vi "mini_test_app.vi"() -> ()   [LabVIEW 2015]
doc: "Mini test app"
uses:
  <vilib>/Utility/error.llb/DialogType.ctl
  Type Definitions/Highway_Data_Control.ctl
panel:
  out "GB ID":string="\r\n" caption="GB Instrument ID"
  out "Hi-Pot ID":string="\r\n" caption="Hi-Pot Instrument ID"
  out "I/F type":string caption="Interface type"
  out "Results GB":string
  out "Status GB":string
  in  "Stop GB":bool
  in  "Start GB":bool
  in  "Stop HiPot":bool
  out "Results HP":string
  in  "Exit Button":bool
  in  "Start HiPot":bool
  out "Status HP":string
  # "Warning. This app is a proof of concept and has no other purpose, \nit is not intended for production. Likewise, it has no error handling. \nUse at your own risk."
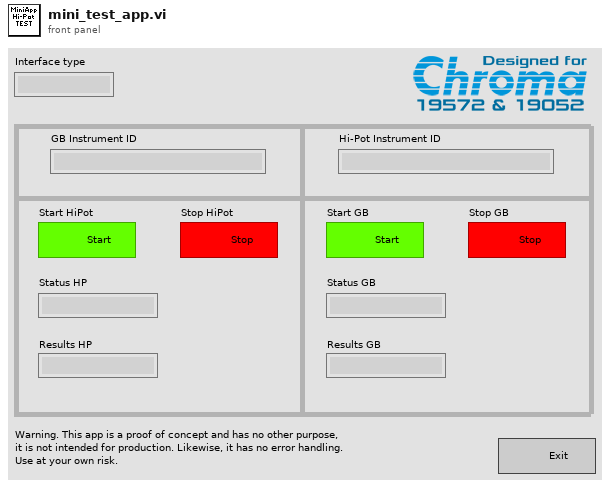
[diagram p1: front panel]
types:
  T1 = typedef "Highway_Data_Control.ctl" = cluster{"Status HP":string, "Results HP":string, "Status GB":string, "Results GB":string}
  T2 = typedef "DialogType.ctl" = u16
  T3 = cluster{"VISA1 Inst ID":string, "VISA2 Inst ID":string, "I/F type":string}
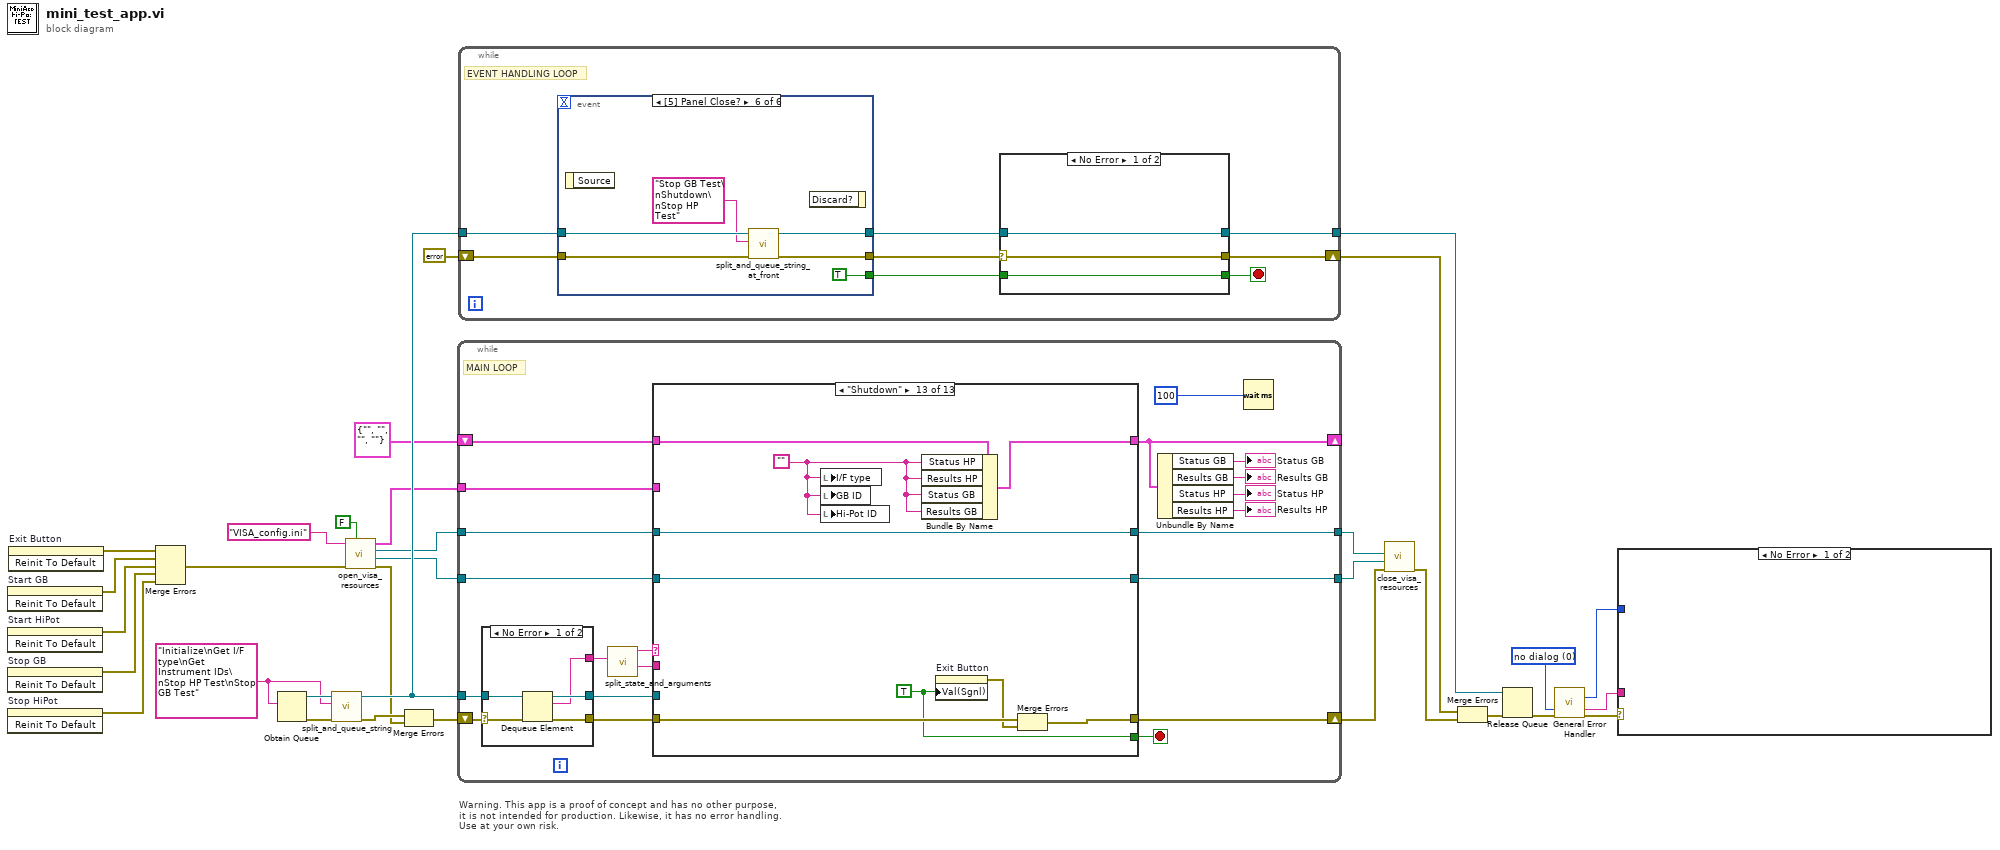
[diagram p0: block diagram]
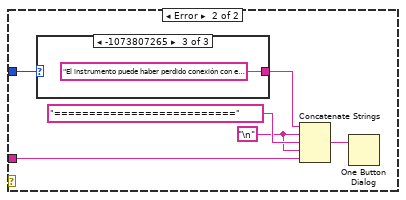
[diagram p2: hidden frame]
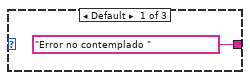
[diagram p3: hidden frame]
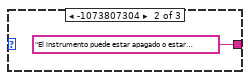
[diagram p4: hidden frame]
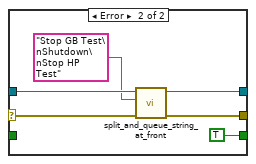
[diagram p5: hidden frame]
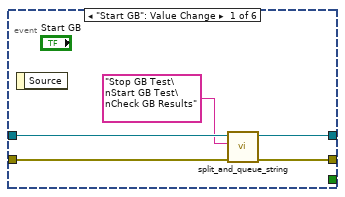
[diagram p6: hidden frame]
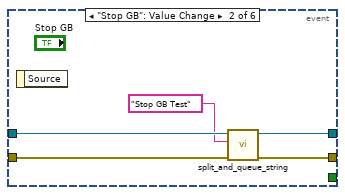
[diagram p7: hidden frame]
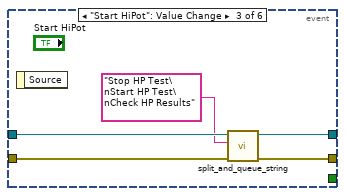
[diagram p8: hidden frame]
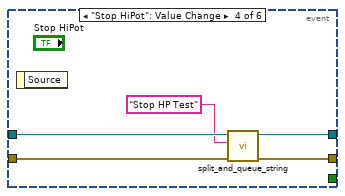
[diagram p9: hidden frame]
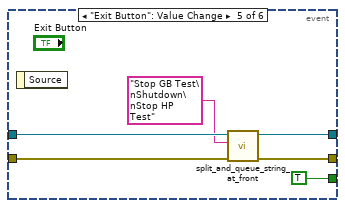
[diagram p10: hidden frame]
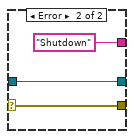
[diagram p11: hidden frame]
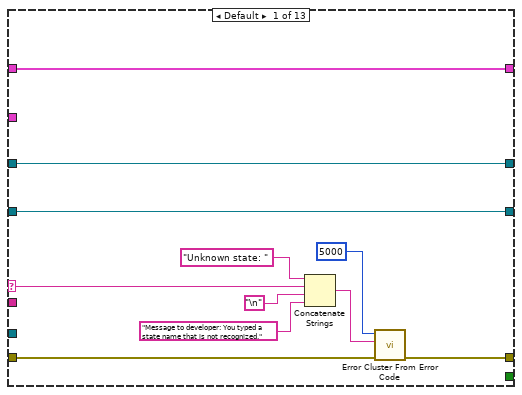
[diagram p12: hidden frame]
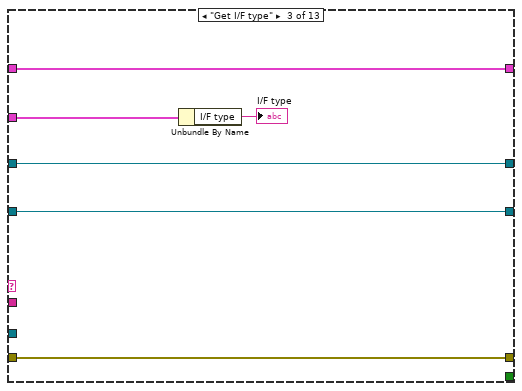
[diagram p14: hidden frame]
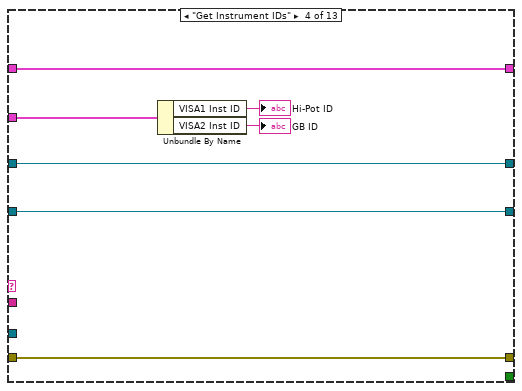
[diagram p15: hidden frame]
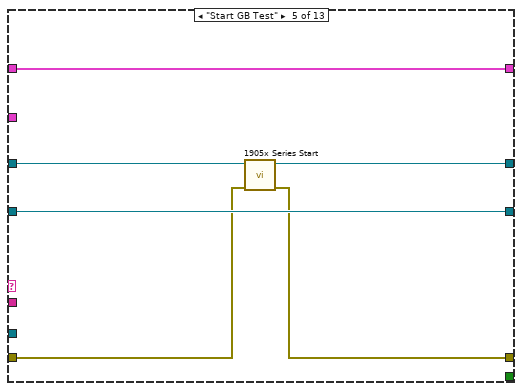
[diagram p16: hidden frame]
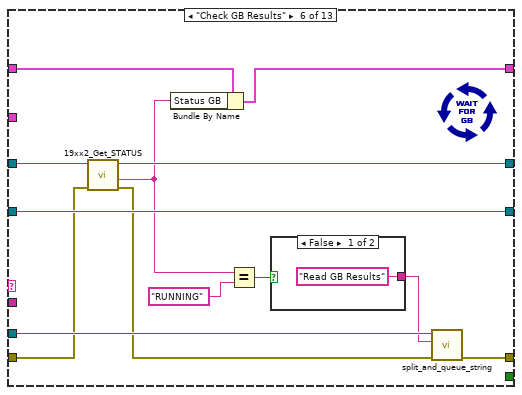
[diagram p17: hidden frame]
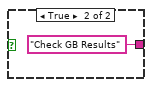
[diagram p18: hidden frame]
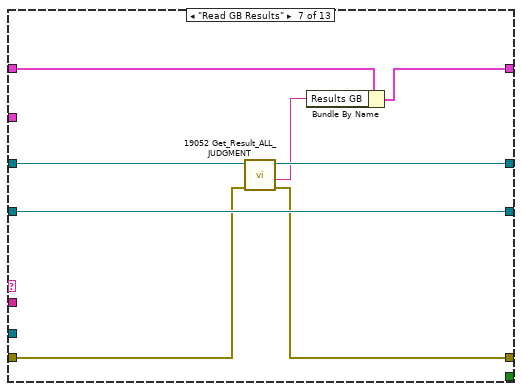
[diagram p19: hidden frame]
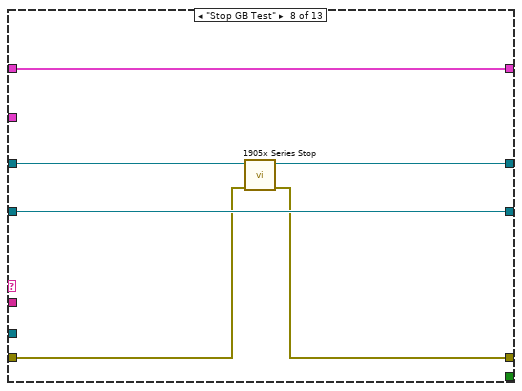
[diagram p20: hidden frame]
diagram:
  w13 = T2 0 items=["no dialog", "OK message", "continue or stop message", "OK message + warnings", "continue/stop + warnings"] ("type of dialog (OK msg:1)")
  w26 = "Initialize\nGet I/F type\nGet Instrument IDs\nStop HP Test\nStop GB Test" ("program string")
  # "Warning. This app is a proof of concept and has no other purpose, \nit is not intended for production. Likewise, it has no error handling. \nUse at your own risk."
  n1 = invoke on="Start GB" class="Bool" method="Reinit To Default"() -> (error out=w5:errorcluster)  [unwired: 3 in, 2 out]
  n2 = invoke on="Start HiPot" class="Bool" method="Reinit To Default"() -> (error out=w4:errorcluster)  [unwired: 3 in, 2 out]
  n3 = invoke on="Stop GB" class="Bool" method="Reinit To Default"() -> (error out=w3:errorcluster)  [unwired: 3 in, 2 out]
  n4 = invoke on="Stop HiPot" class="Bool" method="Reinit To Default"() -> (error out=w2:errorcluster)  [unwired: 3 in, 2 out]
  n5 = invoke on="Exit Button" class="Bool (strict)" method="Reinit To Default"() -> (error out=w7:errorcluster)  [unwired: 3 in, 2 out]
  n6 = Merge Errors(w7, w5, w4, w3, w2) -> (w6:errorcluster)
  n7 = Obtain Queue(element data type=w26) -> (queue out=w32:refnum<queue>, error out=w31:errorcluster)  [unwired: 4 in, 1 out]
  n8 = call "split_and_queue_string.vi"("error in (no error)"=w31, "program string"=w26, "queue in"=w32) -> ("error out"=w25:errorcluster, "queue out"=w24:refnum<queue>)  [unwired: 7 in]
  n9 = call "open_visa_resources.vi"("test mode"=FALSE, "error in (no error)"=w6, "config file in"="VISA_config.ini") -> ("error out"=w17:errorcluster, "VISA resource name for 19052"=w16:refnum<visa-resource-name>, "VISA resource name for 19572"=w9:refnum<visa-resource-name>, "Assgs"=w15:T3)  [unwired: 5 in]
  n10 = Merge Errors(w25, w17) -> (w18:errorcluster)
  n11 = while {
    shift-right: [w51] -> w21
    shift-left: w18 -> [w39]
    tunnel: w24 -> [w40]
    tunnel: w15 -> [w44]
    tunnel: w16 -> [w47]
    tunnel: [w46] -> w22
    tunnel: w9 -> [w43]
    tunnel: [w42] -> w8
    shift-right: [w37] -> _
    shift-left: T1 {"Status HP"="", "Results HP"="", "Status GB"="", "Results GB"=""} -> [w38]
    stop <- w45 stop-if-true
    # "MAIN LOOP"
    n12 = case shown="No Error" w39 {
      selector: w39 -> [w58 w61]
      tunnel: [w57 w61] -> w52
      tunnel: w40 -> [w54 w60]
      tunnel: [w56 w60] -> w41
      tunnel: [w55 "Shutdown"] -> w49
      frame No Error {
        n13 = Dequeue Element(queue=w54, error in (no error)=w58) -> (queue out=w56:refnum<queue>, element=w55:string, error out=w57:errorcluster)  [unwired: 1 in, 1 out]
      }
      frame Error {
      }
    }
    n14 = call "split_state_and_arguments.vi"("String"=w49) -> ("Arguments"=w48:string, "State"=w50:string)  [unwired: 9 in]
    n15 = case shown="\"Shutdown\"" w50 {
      selector: w50 -> [w67 _ _ _ _ _ _ _ _ _ _ _ _]
      tunnel: [w65 w75 w82 w89 w94 w103 w116 w122 w129 w137 w150 w156 w166] -> w51
      tunnel: w52 -> [w66 w75 w82 w89 w93 w106 w117 w123 w127 w140 w152 w158 w168]
      tunnel: w41 -> [_ _ _ _ _ w107 _ _ _ w143 _ _ _]
      tunnel: w48 -> [_ _ _ _ _ _ _ _ _ _ _ _ _]
      tunnel: w47 -> [w72 w76 w81 w88 w95 w108 w118 w124 w128 w141 w153 w159 w164]
      tunnel: [w72 w76 w81 w88 w95 w108 w118 w124 w130 w142 w151 w157 w164] -> w46
      tunnel: [_ _ _ _ _ _ _ _ _ _ _ _ w167] -> w45
      tunnel: w44 -> [_ _ w78 w86 _ _ _ _ _ _ _ _ _]
      tunnel: w43 -> [w63 w74 w80 w87 w92 w100 w115 w121 w126 w134 w149 w155 w163]
      tunnel: [w63 w74 w80 w87 w91 w99 w114 w120 w126 w134 w149 w155 w163] -> w42
      tunnel: w38 -> [w62 w73 w77 w83 w90 w98 w113 w119 w125 w133 w148 w154 w162]
      tunnel: [w62 w73 w77 w83 w90 w97 w112 w119 w125 w132 w147 w154 w161] -> w37
      frame Default {
        n16 = Concatenate Strings("Unknown state: " ("string"), w67, "\n", "Message to developer: You typed a state name that is not recognized.") -> (w69:string)
        n17 = call <vilib>:"Error Cluster From Error Code.vi"("error in (no error)"=w66, "error message (\"\")"=w69, "error code (0)"=5000) -> ("error out"=w65:errorcluster)  [unwired: 6 in]
      }
      frame "Initialize" {
      }
      frame "Get I/F type" {
        n18 = Unbundle By Name(w78) -> ("I/F type"=→"I/F type":string)
      }
      frame "Get Instrument IDs" {
        n19 = Unbundle By Name(w86) -> ("VISA1 Inst ID"=→"Hi-Pot ID":string, "VISA2 Inst ID"=→"GB ID":string)
      }
      frame "Start GB Test" {
        n20 = call "1905x Series Start.vi"("error in (no error)"=w93, "VISA resource in"=w92) -> ("error out"=w94:errorcluster, "VISA resource out"=w91:refnum<visa-resource-name>)  [unwired: 8 in]
      }
      frame "Check GB Results" {
        n21 = call "19xx2_Get_STATUS.vi"("error in (no error)"=w106, "VISA resource in"=w100) -> ("error out"=w104:errorcluster, "Status"=w96:string, "VISA resource out"=w99:refnum<visa-resource-name>)  [unwired: 7 in]
        n22 = Bundle By Name(cluster=w98, "Status GB"=w96) -> (w97:T1)
        n23 = Equal?(x=w96, y="RUNNING") -> (x = y?=w101:bool)
        n24 = case shown="False" w101 {
          tunnel: ["Read GB Results" ("program string") "Check GB Results" ("program string")] -> w102
          frame False {
          }
          frame True {
          }
        }
        n25 = call "split_and_queue_string.vi"("error in (no error)"=w104, "program string"=w102, "queue in"=w107) -> ("error out"=w103:errorcluster)  [unwired: 7 in, 1 out]
      }
      frame "Read GB Results" {
        n26 = call "19052 Get_Result_ALL_JUDGMENT.vi"("error in (no error)"=w117, "VISA resource in"=w115) -> ("error out"=w116:errorcluster, "JUDGMENT"=w111:string, "VISA resource out"=w114:refnum<visa-resource-name>)  [unwired: 7 in]
        n27 = Bundle By Name(cluster=w113, "Results GB"=w111) -> (w112:T1)
      }
      frame "Stop GB Test" {
        n28 = call "1905x Series Stop.vi"("error in (no error)"=w123, "VISA resource in"=w121) -> ("error out"=w122:errorcluster, "VISA resource out"=w120:refnum<visa-resource-name>)  [unwired: 8 in]
      }
      frame "Start HP Test" {
        n29 = call "1905x Series Start.vi"("error in (no error)"=w127, "VISA resource in"=w128) -> ("error out"=w129:errorcluster, "VISA resource out"=w130:refnum<visa-resource-name>)  [unwired: 8 in]
      }
      frame "Check HP Results" {
        n30 = call "19xx2_Get_STATUS.vi"("error in (no error)"=w140, "VISA resource in"=w141) -> ("error out"=w138:errorcluster, "Status"=w131:string, "VISA resource out"=w142:refnum<visa-resource-name>)  [unwired: 7 in]
        n31 = Bundle By Name(cluster=w133, "Status HP"=w131) -> (w132:T1)
        n32 = Equal?(x=w131, y="RUNNING") -> (x = y?=w135:bool)
        n33 = case shown="True" w135 {
          tunnel: ["Read HP Results" ("program string") "Check HP Results" ("program string")] -> w136
          frame False {
          }
          frame True {
          }
        }
        n34 = call "split_and_queue_string.vi"("error in (no error)"=w138, "program string"=w136, "queue in"=w143) -> ("error out"=w137:errorcluster)  [unwired: 7 in, 1 out]
      }
      frame "Read HP Results" {
        n35 = call "19052 Get_Result_ALL_JUDGMENT.vi"("error in (no error)"=w152, "VISA resource in"=w153) -> ("error out"=w150:errorcluster, "JUDGMENT"=w146:string, "VISA resource out"=w151:refnum<visa-resource-name>)  [unwired: 7 in]
        n36 = Bundle By Name(cluster=w148, "Results HP"=w146) -> (w147:T1)
      }
      frame "Stop HP Test" {
        n37 = call "1905x Series Stop.vi"("error in (no error)"=w158, "VISA resource in"=w159) -> ("error out"=w156:errorcluster, "VISA resource out"=w157:refnum<visa-resource-name>)  [unwired: 8 in]
      }
      frame "Shutdown" {
        w160 = ""
        w167 = TRUE
        n38 = local write "I/F type"(w160) -> ()
        n39 = local write "GB ID"(w160) -> ()
        n40 = local write "Hi-Pot ID"(w160) -> ()
        n41 = Bundle By Name(cluster=w162, "Status HP"=w160, "Results HP"=w160, "Status GB"=w160, "Results GB"=w160) -> (w161:T1)
        n42 = property on="Exit Button" class="Bool (strict)"("Val(Sgnl)"=w167) -> (error out=w165:errorcluster)  [unwired: 2 in, 1 out]
        n43 = Merge Errors(w168, w165) -> (w166:errorcluster)
      }
    }
    n44 = Unbundle By Name(w37) -> ("Status GB"=→"Status GB":string, "Results GB"=→"Results GB":string, "Status HP"=→"Status HP":string, "Results HP"=→"Results HP":string)
    n45 = Wait (ms)(milliseconds to wait=u32 100) -> ()  [unwired: 1 out]
  }
  n46 = while {
    tunnel: w24 -> [w175]
    tunnel: [w171] -> w27
    shift-right: [w174] -> w30
    shift-left: errorcluster {"status"=FALSE, "code"=0, "source"=""} ("error constant") -> [w176]
    stop <- w172 stop-if-true
    # "EVENT HANDLING LOOP"
    n47 = event shown="[5] Panel Close?" {
      selector: _ -> [_ _ _ _ _ _]
      dyn-events: _ -> [_ _ _ _ _ _]
      timeout: _ -> [_ _ _ _ _ _]
      tunnel: w175 -> [w188 w192 w200 w203 w208 w217]
      tunnel: w176 -> [w187 w194 w199 w205 w207 w215]
      tunnel: [w189 w195 w198 w204 w209 w214] -> w169
      tunnel: [_ _ _ _ TRUE TRUE] -> w173
      tunnel: [w190 w193 w196 w202 w210 w216] -> w170
      event "Start GB": Value Change {
        n48 = event-data() -> ()  [unwired: 1 in, 1 out]
        n49 = call "split_and_queue_string.vi"("error in (no error)"=w187, "program string"="Stop GB Test\nStart GB Test\nCheck GB Results", "queue in"=w188) -> ("error out"=w189:errorcluster, "queue out"=w190:refnum<queue>)  [unwired: 7 in]
      }
      event "Stop GB": Value Change {
        n50 = event-data() -> ()  [unwired: 1 in, 1 out]
        n51 = call "split_and_queue_string.vi"("error in (no error)"=w194, "program string"="Stop GB Test", "queue in"=w192) -> ("error out"=w195:errorcluster, "queue out"=w193:refnum<queue>)  [unwired: 7 in]
      }
      event "Start HiPot": Value Change {
        n52 = event-data() -> ()  [unwired: 1 in, 1 out]
        n53 = call "split_and_queue_string.vi"("error in (no error)"=w199, "program string"="Stop HP Test\nStart HP Test\nCheck HP Results", "queue in"=w200) -> ("error out"=w198:errorcluster, "queue out"=w196:refnum<queue>)  [unwired: 7 in]
      }
      event "Stop HiPot": Value Change {
        n54 = event-data() -> ()  [unwired: 1 in, 1 out]
        n55 = call "split_and_queue_string.vi"("error in (no error)"=w205, "program string"="Stop HP Test", "queue in"=w203) -> ("error out"=w204:errorcluster, "queue out"=w202:refnum<queue>)  [unwired: 7 in]
      }
      event "Exit Button": Value Change {
        n56 = event-data() -> ()  [unwired: 1 in, 1 out]
        n57 = call "split_and_queue_string_at_front.vi"("error in (no error)"=w207, "program string"="Stop GB Test\nShutdown\nStop HP Test", "queue in"=w208) -> ("error out"=w209:errorcluster, "queue out"=w210:refnum<queue>)  [unwired: 7 in]
      }
      event Panel Close? {
        n58 = event-data() -> ()  [unwired: 1 in, 1 out]
        n59 = call "split_and_queue_string_at_front.vi"("error in (no error)"=w215, "program string"="Stop GB Test\nShutdown\nStop HP Test", "queue in"=w217) -> ("error out"=w214:errorcluster, "queue out"=w216:refnum<queue>)  [unwired: 7 in]
        n60 = event-data() -> ()  [unwired: 2 in, 1 out]
      }
    }
    n61 = case shown="No Error" w169 {
      selector: w169 -> [w179 w184]
      tunnel: [w179 w183] -> w174
      tunnel: w173 -> [w178 _]
      tunnel: [w178 TRUE] -> w172
      tunnel: [w177 w182] -> w171
      tunnel: w170 -> [w177 w181]
      frame No Error {
      }
      frame Error {
        n62 = call "split_and_queue_string_at_front.vi"("error in (no error)"=w184, "program string"="Stop GB Test\nShutdown\nStop HP Test", "queue in"=w181) -> ("error out"=w183:errorcluster, "queue out"=w182:refnum<queue>)  [unwired: 7 in]
      }
    }
  }
  n63 = call "close_visa_resources.vi"("error in (no error)"=w21, "VISA resource name in 2"=w22, "VISA resource name in 1"=w8) -> ("error out"=w20:errorcluster)  [unwired: 8 in]
  n64 = Merge Errors(w30, w20) -> (w29:errorcluster)
  n65 = Release Queue(queue=w27, error in (no error)=w29) -> (error out=w28:errorcluster)  [unwired: 1 in, 2 out]
  n66 = call <vilib>:"General Error Handler.vi"("type of dialog (OK msg:1)"=w13, "error in (no error)"=w28) -> ("code out"=w11:i32, "message"=w10:string, "error out"=w12:errorcluster)  [unwired: 9 in, 2 out]
  n67 = case shown="No Error" w12 {
    tunnel: w11 -> [_ w223]
    tunnel: w10 -> [_ w221]
    frame No Error {
    }
    frame Error {
      w218 = "\n"
      n68 = case shown="-1073807265" w223 {
        tunnel: ["Error no contemplado " "El instrumento puede estar apagado o estar reinicinado." "El instrumento puede haber perdido conexión con el host."] -> w222
        frame Default {
        }
        frame -1073807304 {
        }
        frame -1073807265 {
        }
      }
      n69 = Concatenate Strings(w222, w218, "==========================", w218, w221) -> (w220:string)
      n70 = One Button Dialog(message=w220) -> ()  [unwired: 1 in, 1 out]
    }
  }
